vi "MoveForward.vi"(9 "Inches Forward":dbl=26.0, 10 "right enconder":string="My Encoder RefNum", 11 "left enconder":string="My Encoder RefNum") -> ()   [LabVIEW 2019]
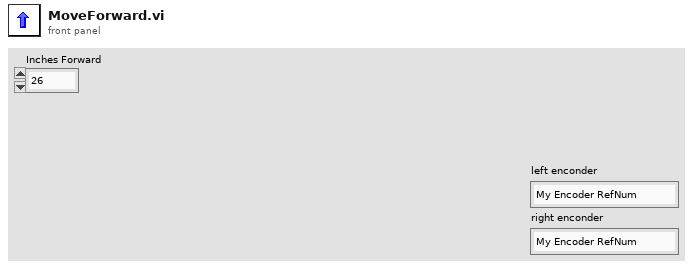
[diagram p1: front panel]
types:
  T1 = typedef "WPI_EncoderDevRef.ctl" = cluster{"DevStatus":errorcluster, "EncoderIndex":T2, "CounterIndex":T3, "DistancePerCount":dbl, "Decoding Type":T4}
  T2 = typedef "FPGA_EncoderIdx.ctl" = enum8{"Enc 0", "Enc 1", "Enc 2", "Enc 3", "Enc 4", "Enc 5", "Enc 6", "Enc 7", "Invalid"}
  T3 = typedef "FPGA_CounterCtrSystemIndex.ctl" = enum8{"Ctr 0", "Ctr 1", "Ctr 2", "Ctr 3", "Ctr 4", "Ctr 5", "Ctr 6", "Ctr 7", "Invalid"}
  T4 = typedef "WPI_EncoderType.ctl" = enum16{"1x", "2x", "4x"}
  T5 = typedef "WPI_RobotDriveDevRef.ctl" = cluster{"DevStatus":errorcluster, "Motors[]":T6[], "Square Inputs":bool, "Max Output":dbl}
  T6 = typedef "WPI_MotorControlDeviceRef.ctl" = cluster{"DeviceStatus":errorcluster, "Type":T7, "PWM":cluster{"PWM Channel":T8, "DeadBand":T9}, "CAN":cluster{"Device Number":u8, "SetOutput VI Ref":variant, "GetOutput VI Ref":variant, "Enable VI Ref":variant, "Disable VI Ref":variant, "Data":variant}, "Invert":bool, "DIO PWM":cluster{"PWM \"Enable\" Channel":T8, "DIOChannel":T10, "PWM Rate":dbl}}
  T7 = typedef "WPI_MotorControlType.ctl" = enum16{"PWM", "CAN", "DIO PWM"}
  T8 = typedef "FPGA_DIOPWMChannel.ctl" = enum8{"PWM 0", "PWM 1", "PWM 2", "PWM 3", "PWM 4", "PWM 5", "PWM 6", "PWM 7", "PWM 8", "PWM 9", "PWM MXP 0", "PWM MXP 1", "PWM MXP 2", "PWM MXP 3", "PWM MXP 4", "PWM MXP 5", "PWM MXP 6", "PWM MXP 7", "PWM MXP 8", "PWM MXP 9", "Invalid"}
  T9 = typedef "WPI_PWMDeadband.ctl" = cluster{"Name":string, "maxPositivePwm":i32, "minPositivePwm":i32, "centerPwm":i32, "maxNegativePwm":i32, "minNegativePwm":i32, "angularRange":u16}
  T10 = typedef "FPGA_DIOChannel.ctl" = enum8{"DIO 0", "DIO 1", "DIO 2", "DIO 3", "DIO 4", "DIO 5", "DIO 6", "DIO 7", "DIO 8", "DIO 9", "DIO MXP 0", "DIO MXP 1", "DIO MXP 2", "DIO MXP 3", "DIO MXP 4", "DIO MXP 5", "DIO MXP 6", "DIO MXP 7", "DIO MXP 8", "DIO MXP 9", "DIO MXP 10", "DIO MXP 11", "DIO MXP 12", "DIO MXP 13", "DIO MXP 14", "DIO MXP 15", "SPI Port CS1", "SPI Port CS2", "SPI Port CS3", "SPI Port MISO", "SPI Port MOSI", "Invalid"}
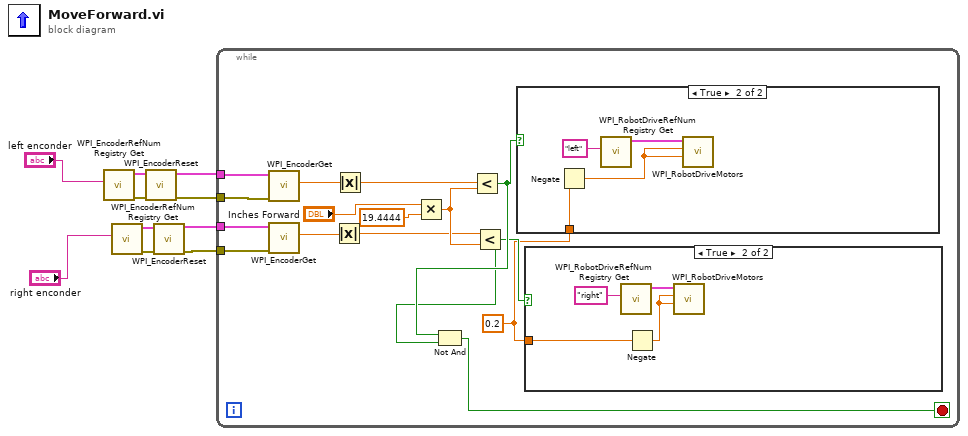
[diagram p0: block diagram]
diagram:
  n1 = call <vilib>:"WPI_EncoderRefNum Registry Get.vi"("refnum name"="left enconder") -> ("error out"=w9:errorcluster, "EncoderDevRef"=w10:T1)  [unwired: 9 in]
  n2 = call <vilib>:"WPI_EncoderRefNum Registry Get.vi"("refnum name"="right enconder") -> ("error out"=w7:errorcluster, "EncoderDevRef"=w8:T1)  [unwired: 9 in]
  n3 = call <vilib>:"WPI_EncoderReset.vi"("error in (no error)"=w9, "EncoderDevRef"=w10) -> ("error out"=w5:errorcluster, "EncoderDevRef"=w6:T1)  [unwired: 8 in]
  n4 = call <vilib>:"WPI_EncoderReset.vi"("error in (no error)"=w7, "EncoderDevRef"=w8) -> ("error out"=w3:errorcluster, "EncoderDevRef"=w4:T1)  [unwired: 8 in]
  n5 = while {
    tunnel: w6 -> [w25]
    tunnel: w5 -> [w24]
    tunnel: w4 -> [w23]
    tunnel: w3 -> [w22]
    stop <- w12 stop-if-true
    w11 = 0.2 ("x")
    n6 = call <vilib>:"WPI_EncoderGet.vi"("error in (no error)"=w24, "EncoderDevRef"=w25) -> ("Distance"=w20:dbl)  [unwired: 4 in, 5 out]
    n7 = call <vilib>:"WPI_EncoderGet.vi"("error in (no error)"=w22, "EncoderDevRef"=w23) -> ("Distance"=w21:dbl)  [unwired: 4 in, 5 out]
    n8 = Absolute Value(x=w21) -> (abs(x)=w15:dbl)
    n9 = Absolute Value(x=w20) -> (abs(x)=w19:dbl)
    n10 = Multiply(x="Inches Forward", y=19.4444) -> (x*y=w16:dbl)
    n11 = Less?(x=w19, y=w16) -> (x < y?=w14:bool)
    n12 = Less?(x=w15, y=w16) -> (x < y?=w13:bool)
    n13 = Not And(1:w13, 2:w14) -> (0:w12:bool)
    n14 = case shown="True" w14 {
      tunnel: w11 -> [_ w30]
      frame False {
      }
      frame True {
        n15 = Negate(x=w30) -> (-x=w33:dbl)
        n16 = call <vilib>:"WPI_RobotDriveRefNum Registry Get.vi"("refnum name"="left") -> ("RobotDriveDevRef"=w31:T5)  [unwired: 1 in, 9 out]
        n17 = call <vilib>:"WPI_RobotDriveMotors.vi"("RightSpeed"=w33, "LeftSpeed"=w33, "RobotDriveDevRef"=w31) -> ()  [unwired: 6 in, 3 out]
      }
    }
    n18 = case shown="True" w13 {
      tunnel: w11 -> [_ w26]
      frame False {
      }
      frame True {
        n19 = call <vilib>:"WPI_RobotDriveRefNum Registry Get.vi"("refnum name"="right") -> ("RobotDriveDevRef"=w28:T5)  [unwired: 1 in, 9 out]
        n20 = Negate(x=w26) -> (-x=w29:dbl)
        n21 = call <vilib>:"WPI_RobotDriveMotors.vi"("RightSpeed"=w29, "LeftSpeed"=w29, "RobotDriveDevRef"=w28) -> ()  [unwired: 6 in, 3 out]
      }
    }
  }
